vi "Car Wash.vi"() -> ()   [LabVIEW 2025]
uses:
  Controls/Car Wash Indicators.ctl
  Controls/Wash Options.ctl
  Controls/Controls.ctl
panel:
  in  "Start":bool
  out "Elapsed Time":dbl format="%0.2f"
  in  "stop":bool
  out "Wash Entry":bool
  in  "Wash Options":T1
  in  "Car Position Slider":u8(slide) max=3 scale=0.0..4.0
  out "Car Wash Indicators":T2
  # "Entry Console"
  # "Car Wash Display"
  # "Car Position Simulation"
  # "Pre-Soak\nH-P Wash\nL-P Wax\nSpot Free Rinse"
  # "Underbody Wash\nBug Remover"
  # "Tire Shine\nAir Dry"
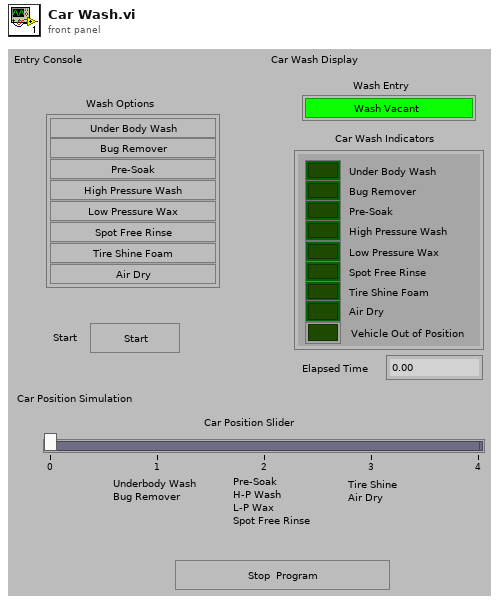
[diagram p1: front panel]
types:
  T1 = typedef "Wash Options.ctl" = cluster{"Underbody Wash":bool, "Bug Remover":bool, "Pre-Soak":bool, "High Pressure Wash":bool, "Low Pressure Wax":bool, "Spot Free Rinse":bool, "Tire Shine Foam":bool, "Air Dry":bool}
  T2 = typedef "Car Wash Indicators.ctl" = cluster{"Under Body Wash":bool, "Bug Remover":bool, "Pre-Soak":bool, "High Pressure Wash":bool, "Low Pressure Wax":bool, "Spot Free Rinse":bool, "Tire Shine Foam":bool, "Air Dry":bool, "Vehicle Out of Position":bool}
  T3 = typedef "Controls.ctl" = enum16{"Initialization", "Wait For Start", "Car Wash Setup", "Under Body Wash", "Bug Remover", "Pre-Soak", "High Pressure Wash", "Low Pressure Wash", "Spot Free Rinse", "Tire Shine Foam", "Air Dry", "Exit"}
  T4 = enum8{"Enabled", "Disabled", "Disabled and Grayed Out"}
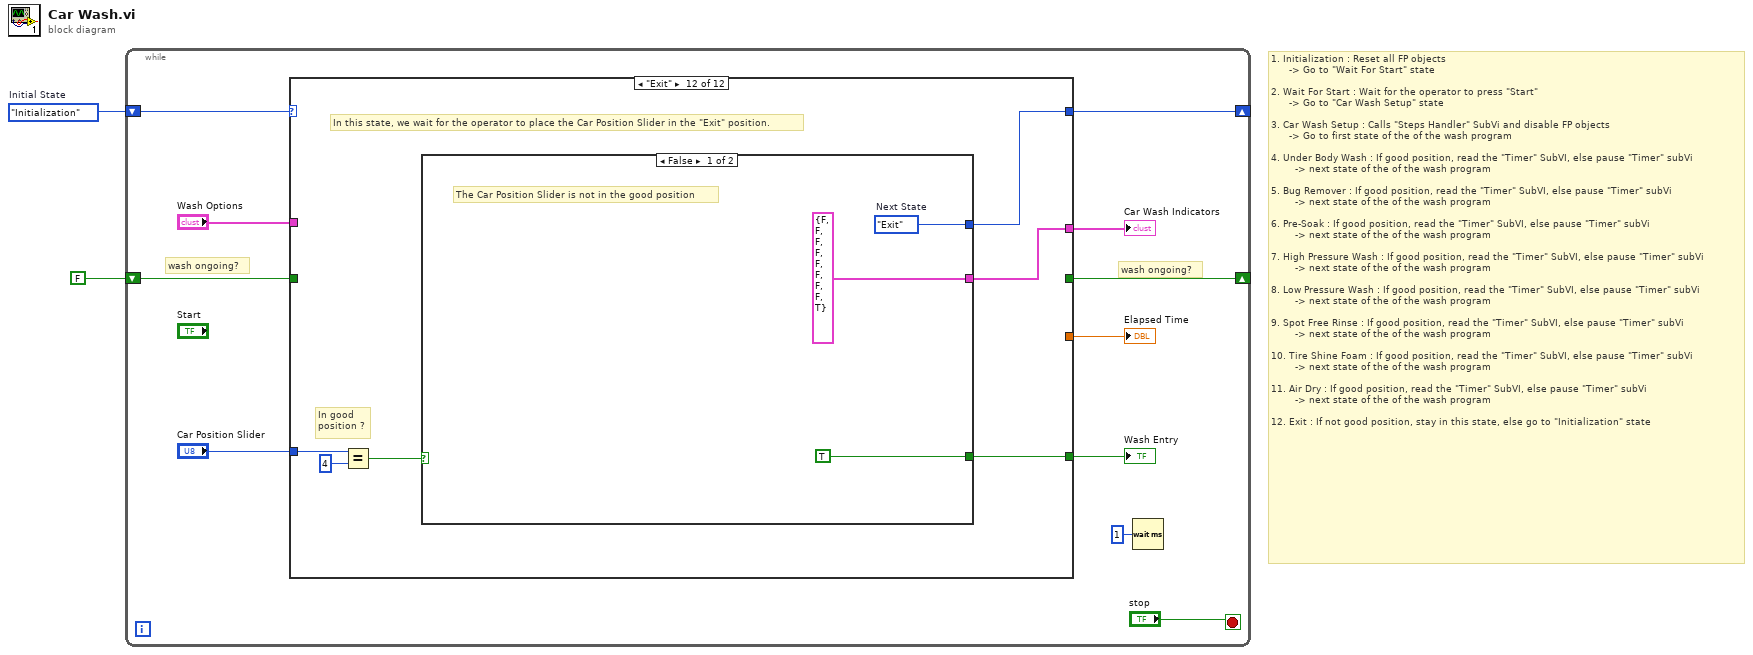
[diagram p0: block diagram]
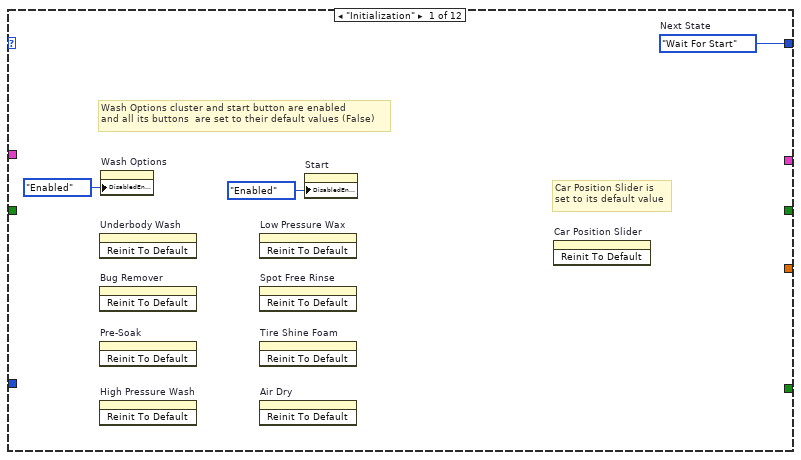
[diagram p2: hidden frame]
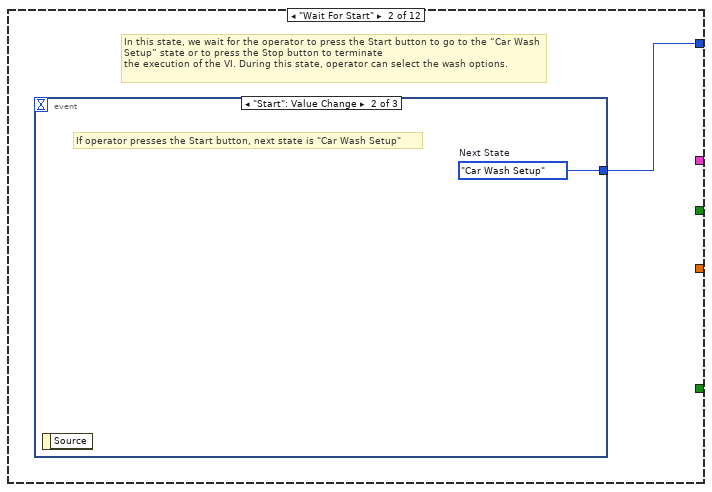
[diagram p3: hidden frame]
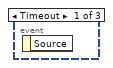
[diagram p4: hidden frame]
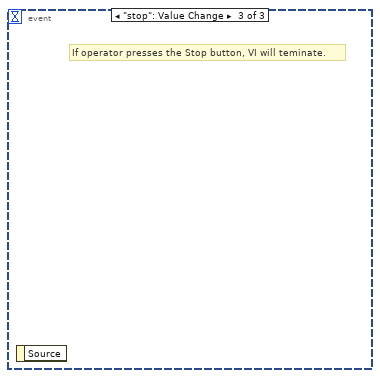
[diagram p5: hidden frame]
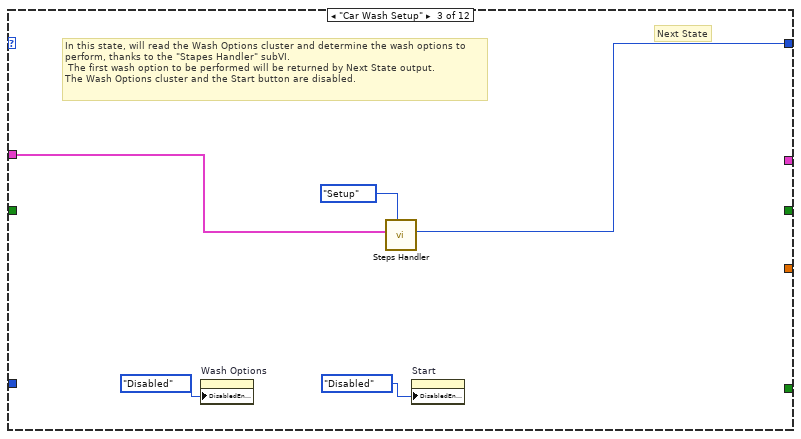
[diagram p6: hidden frame]
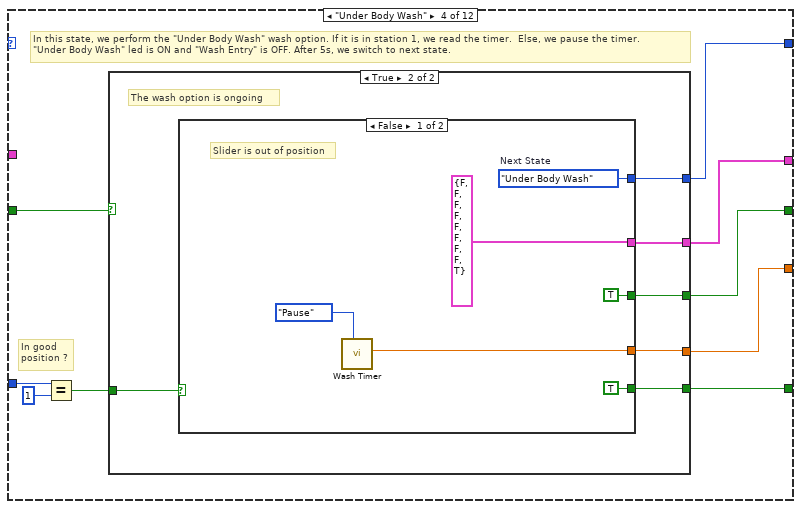
[diagram p7: hidden frame]
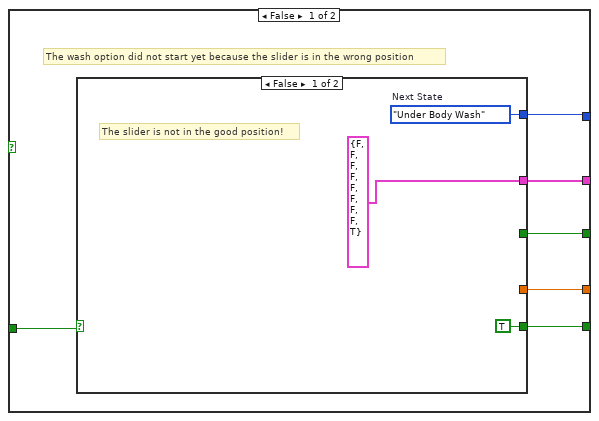
[diagram p8: hidden frame]
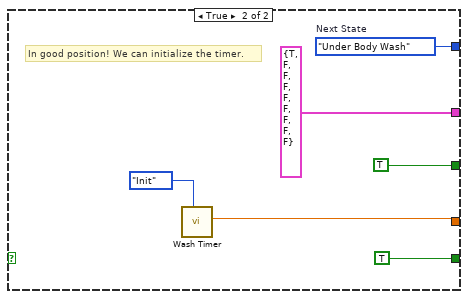
[diagram p9: hidden frame]
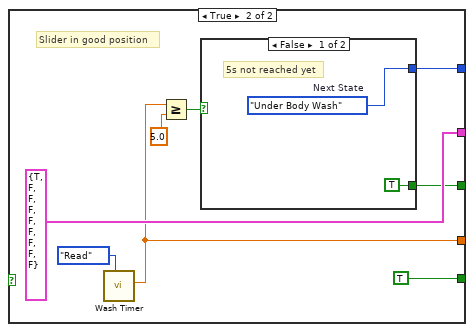
[diagram p10: hidden frame]
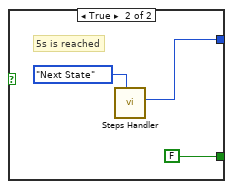
[diagram p11: hidden frame]
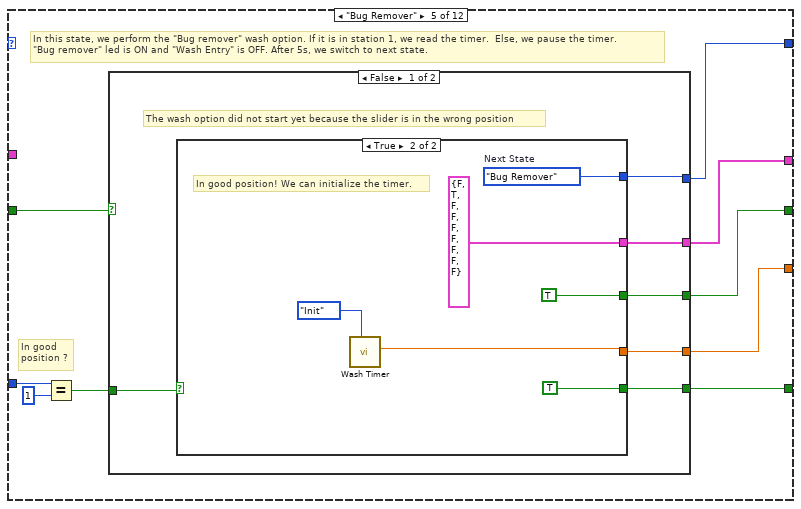
[diagram p12: hidden frame]
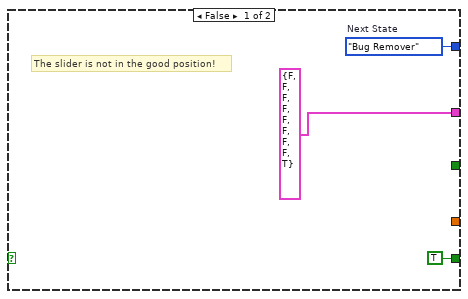
[diagram p13: hidden frame]
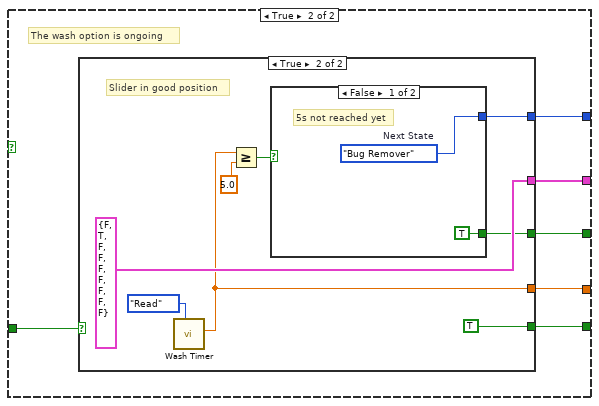
[diagram p14: hidden frame]
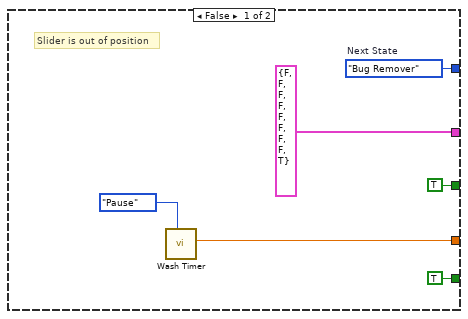
[diagram p15: hidden frame]
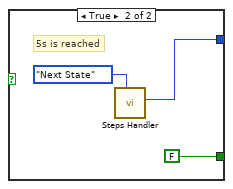
[diagram p16: hidden frame]
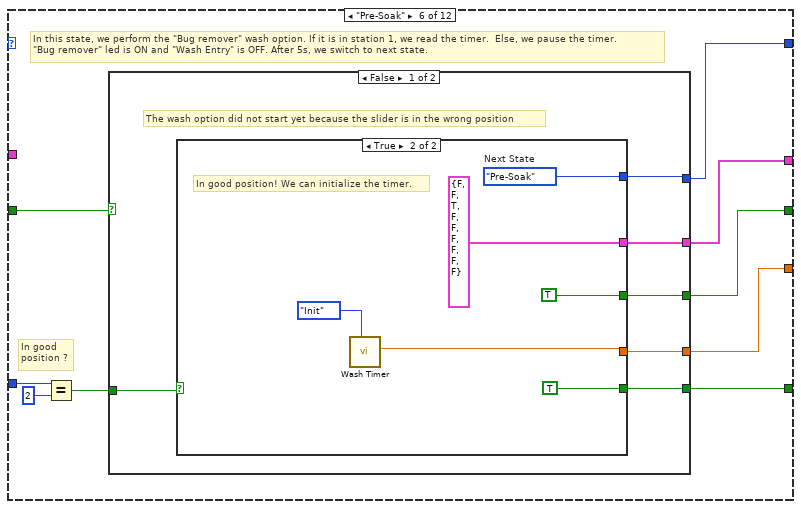
[diagram p17: hidden frame]
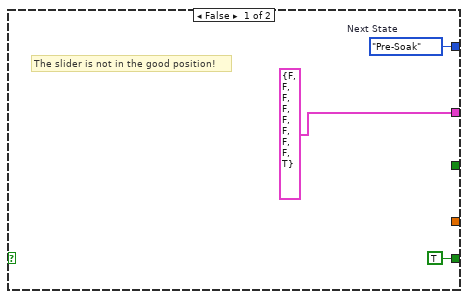
[diagram p18: hidden frame]
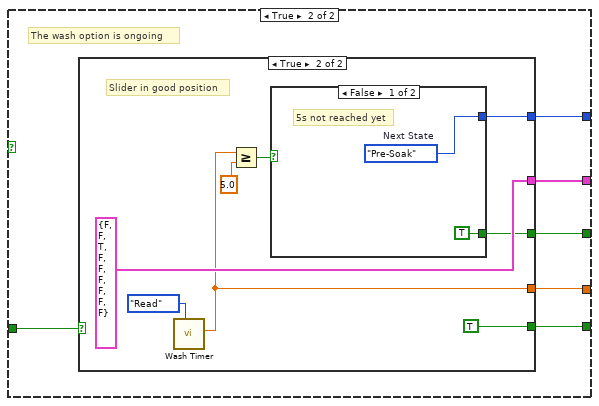
[diagram p19: hidden frame]
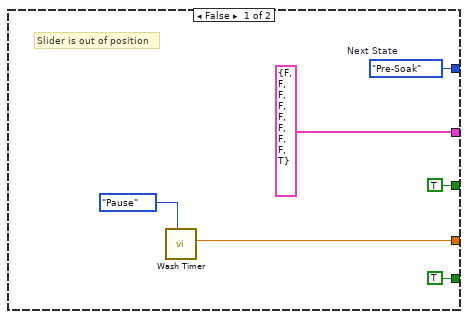
[diagram p20: hidden frame]
diagram:
  w2 = Controls."Initialization"  # Initial State
  # "1. Initialization : Reset all FP objects\n      -> Go to \"Wait For Start\" state\n\n2. Wait For Start : Wait for the operator to press \"Start\"\n      -> Go to \"Car Wash Setup\" state\n\n3. Car Wash Setup : Calls \"Steps Handler\" SubVi and disable FP objects \n      -> Go to first state of the of the wash program \n\n4. Under Body Wash : If good position, read the \"Timer\" SubVI, else pause \"Timer\" subVi\n        -> next state of the of the wash program\n\n5. Bug Remover : If good position, read the \"Timer\" SubVI, else pause \"Timer\" subVi\n        -> next state of the of the wash program\n\n6. Pre-Soak : If good position, read the \"Timer\" SubVI, else pause \"Timer\" subVi\n        -> next state of the of the wash program\n\n7. High Pressure Wash : If good position, read the \"Timer\" SubVI, else pause \"Timer\" subVi\n        -> next state of the of the wash program\n\n8. Low Pressure Wash : If good position, read the \"Timer\" SubVI, else pause \"Timer\" subVi\n        -> next state of the of the wash program\n\n9. Spot Free Rinse : If good position, read the \"Timer\" SubVI, else pause \"Timer\" subVi\n        -> next state of the of the wash program\n\n10. Tire Shine Foam : If good position, read the \"Timer\" SubVI, else pause \"Timer\" subVi\n        -> next state of the of the wash program\n\n11. Air Dry : If good position, read the \"Timer\" SubVI, else pause \"Timer\" subVi\n        -> next state of the of the wash program\n\n12. Exit : If not good position, stay in this state, else go to \"Initialization\" state"
  n1 = while {
    shift-right: [w10] -> _
    shift-left: w2 -> [w13]
    shift-right: [w6] -> _
    shift-left: FALSE -> [w7]
    stop <- "stop" stop-if-true
    # "wash ongoing?"
    # "wash ongoing?"
    n2 = case shown="\"Exit\"" w13 {
      tunnel: [w15 w17 w21 w27 w76 w125 w174 w223 w272 w321 w370 w418] -> w10
      tunnel: "Wash Options" -> [_ _ w22 _ _ _ _ _ _ _ _ _]
      tunnel: "Car Position Slider" -> [_ _ _ w32 w81 w130 w179 w228 w277 w326 w375 w420]
      tunnel: w7 -> [_ _ _ w30 w79 w128 w177 w226 w275 w324 w373 _]
      tunnel: [_ _ _ w28 w77 w126 w175 w224 w273 w322 w371 _] -> w6
      tunnel: [_ _ _ w26 w75 w124 w173 w222 w271 w320 w369 w417] -> w5
      tunnel: [_ _ _ w25 w74 w123 w172 w221 w270 w319 w368 _] -> w4
      tunnel: [_ _ _ w24 w73 w122 w171 w220 w269 w318 w367 w416] -> w3
      frame "Initialization" {
        w15 = Controls."Wait For Start"  # Next State
        # "Car Position Slider is \nset to its default value"
        # "Wash Options cluster and start button are enabled \nand all its buttons  are set to their default values (False)"
        n3 = invoke on="Underbody Wash" class="Bool (strict)" method="Reinit To Default"() -> ()  [unwired: 3 in, 3 out]
        n4 = invoke on="Bug Remover" class="Bool (strict)" method="Reinit To Default"() -> ()  [unwired: 3 in, 3 out]
        n5 = invoke on="Pre-Soak" class="Bool (strict)" method="Reinit To Default"() -> ()  [unwired: 3 in, 3 out]
        n6 = invoke on="High Pressure Wash" class="Bool (strict)" method="Reinit To Default"() -> ()  [unwired: 3 in, 3 out]
        n7 = property on="Wash Options" class="Clust (strict)"("DisabledEnum"=T4."Enabled" ("Disabled")) -> ()  [unwired: 2 in, 2 out]
        n8 = invoke on="Low Pressure Wax" class="Bool (strict)" method="Reinit To Default"() -> ()  [unwired: 3 in, 3 out]
        n9 = invoke on="Spot Free Rinse" class="Bool (strict)" method="Reinit To Default"() -> ()  [unwired: 3 in, 3 out]
        n10 = invoke on="Tire Shine Foam" class="Bool (strict)" method="Reinit To Default"() -> ()  [unwired: 3 in, 3 out]
        n11 = invoke on="Air Dry" class="Bool (strict)" method="Reinit To Default"() -> ()  [unwired: 3 in, 3 out]
        n12 = property on="Start" class="Bool"("DisabledEnum"=T4."Enabled" ("Disabled")) -> ()  [unwired: 2 in, 2 out]
        n13 = invoke on="Car Position Slider" class="Slide (strict)" method="Reinit To Default"() -> ()  [unwired: 3 in, 3 out]
      }
      frame "Wait For Start" {
        # "In this state, we wait for the operator to press the Start button to go to the “Car Wash Setup” state or to press the Stop button to terminate \nthe execution of the VI. During this state, operator can select the wash options."
        n14 = event shown="[1] \"Start\": Value Change" {
          selector: _ -> [_ _ _]
          dyn-events: _ -> [_ _ _]
          timeout: _ -> [_ _ _]
          tunnel: [_ w18 _] -> w17
          event Timeout {
            n15 = event-data() -> ()  [unwired: 1 in, 1 out]
          }
          event "Start": Value Change {
            w18 = Controls."Car Wash Setup"  # Next State
            # "If operator presses the Start button, next state is \"Car Wash Setup\""
            n16 = event-data() -> ()  [unwired: 1 in, 1 out]
          }
          event "stop": Value Change {
            # "If operator presses the Stop button, VI will teminate."
            n17 = event-data() -> ()  [unwired: 1 in, 1 out]
          }
        }
      }
      frame "Car Wash Setup" {
        # "In this state, will read the Wash Options cluster and determine the wash options to perform, thanks to the \"Stapes Handler\" subVI.\n The first wash option to be performed will be returned by Next State output.\nThe Wash Options cluster and the Start button are disabled."
        # "Next State"
        n18 = property on="Wash Options" class="Clust (strict)"("DisabledEnum"=T4."Disabled" ("Disabled")) -> ()  [unwired: 2 in, 2 out]
        n19 = call "Steps Handler.vi"("Operation"=enum16{"Setup", "Next State"}."Setup", "Wash Options"=w22) -> ("Next State"=w21:T3)  [unwired: 9 in]
        n20 = property on="Start" class="Bool"("DisabledEnum"=T4."Disabled" ("Disabled")) -> ()  [unwired: 2 in, 2 out]
      }
      frame "Under Body Wash" {
        # "In good \nposition ?"
        # "In this state, we perform the \"Under Body Wash\" wash option. If it is in station 1, we read the timer.  Else, we pause the timer. \n\"Under Body Wash\" led is ON and \"Wash Entry\" is OFF. After 5s, we switch to next state."
        n21 = Equal?(x=w32, y=u8 1) -> (x = y?=w29:bool)
        n22 = case shown="True" w30 {
          tunnel: w29 -> [w38 w53]
          tunnel: [w37 w48] -> w28
          tunnel: [w36 w49] -> w27
          tunnel: [w35 w50] -> w26
          tunnel: [w34 w52] -> w25
          tunnel: [w33 w51] -> w24
          frame False {
            # "The wash option did not start yet because the slider is in the wrong position"
            n23 = case shown="False" w38 {
              tunnel: [_ TRUE] -> w37
              tunnel: [w41 w46] -> w36
              tunnel: [T2 {"Under Body Wash"=FALSE, "Bug Remover"=FALSE, "Pre-Soak"=FALSE, "High Pressure Wash"=FALSE, "Low Pressure Wax"=FALSE, "Spot Free Rinse"=FALSE, "Tire Shine Foam"=FALSE, "Air Dry"=FALSE, "Vehicle Out of Position"=TRUE} ("Car Wash Indicators") T2 {"Under Body Wash"=TRUE, "Bug Remover"=FALSE, "Pre-Soak"=FALSE, "High Pressure Wash"=FALSE, "Low Pressure Wax"=FALSE, "Spot Free Rinse"=FALSE, "Tire Shine Foam"=FALSE, "Air Dry"=FALSE, "Vehicle Out of Position"=FALSE} ("Car Wash Indicators")] -> w35
              tunnel: [_ w43] -> w34
              tunnel: [TRUE TRUE] -> w33
              frame False {
                w41 = Controls."Under Body Wash"  # Next State
                # "The slider is not in the good position!"
              }
              frame True {
                w46 = Controls."Under Body Wash"  # Next State
                # "In good position! We can initialize the timer."
                n24 = call "Wash Timer.vi"("Operation"=enum16{"Init", "Read", "Pause"}."Init") -> ("count"=w43:dbl)  [unwired: 10 in]
              }
            }
          }
          frame True {
            # "The wash option is ongoing"
            n25 = case shown="False" w53 {
              tunnel: [w58 w64] -> w52
              tunnel: [TRUE TRUE] -> w51
              tunnel: [T2 {"Under Body Wash"=FALSE, "Bug Remover"=FALSE, "Pre-Soak"=FALSE, "High Pressure Wash"=FALSE, "Low Pressure Wax"=FALSE, "Spot Free Rinse"=FALSE, "Tire Shine Foam"=FALSE, "Air Dry"=FALSE, "Vehicle Out of Position"=TRUE} ("Car Wash Indicators") T2 {"Under Body Wash"=TRUE, "Bug Remover"=FALSE, "Pre-Soak"=FALSE, "High Pressure Wash"=FALSE, "Low Pressure Wax"=FALSE, "Spot Free Rinse"=FALSE, "Tire Shine Foam"=FALSE, "Air Dry"=FALSE, "Vehicle Out of Position"=FALSE} ("Car Wash Indicators")] -> w50
              tunnel: [w57 w61] -> w49
              tunnel: [TRUE w60] -> w48
              frame False {
                w57 = Controls."Under Body Wash"  # Next State
                # "Slider is out of position"
                n26 = call "Wash Timer.vi"("Operation"=enum16{"Init", "Read", "Pause"}."Pause") -> ("count"=w58:dbl)  [unwired: 10 in]
              }
              frame True {
                # "Slider in good position"
                n27 = call "Wash Timer.vi"("Operation"=enum16{"Init", "Read", "Pause"}."Read") -> ("count"=w64:dbl)  [unwired: 10 in]
                n28 = Greater Or Equal?(x=w64, y=5.0) -> (x >= y?=w62:bool)
                n29 = case shown="False" w62 {
                  tunnel: [w69 w71] -> w61
                  tunnel: [TRUE FALSE] -> w60
                  frame False {
                    w69 = Controls."Under Body Wash"  # Next State
                    # "5s not reached yet"
                  }
                  frame True {
                    # "5s is reached"
                    n30 = call "Steps Handler.vi"("Operation"=enum16{"Setup", "Next State"}."Next State") -> ("Next State"=w71:T3)  [unwired: 10 in]
                  }
                }
              }
            }
          }
        }
      }
      frame "Bug Remover" {
        # "In good \nposition ?"
        # "In this state, we perform the \"Bug remover\" wash option. If it is in station 1, we read the timer.  Else, we pause the timer. \n\"Bug remover\" led is ON and \"Wash Entry\" is OFF. After 5s, we switch to next state."
        n31 = Equal?(x=w81, y=u8 1) -> (x = y?=w78:bool)
        n32 = case shown="False" w79 {
          tunnel: w78 -> [w87 w102]
          tunnel: [w86 w97] -> w77
          tunnel: [w85 w98] -> w76
          tunnel: [w84 w99] -> w75
          tunnel: [w83 w101] -> w74
          tunnel: [w82 w100] -> w73
          frame False {
            # "The wash option did not start yet because the slider is in the wrong position"
            n33 = case shown="True" w87 {
              tunnel: [_ TRUE] -> w86
              tunnel: [w90 w95] -> w85
              tunnel: [T2 {"Under Body Wash"=FALSE, "Bug Remover"=FALSE, "Pre-Soak"=FALSE, "High Pressure Wash"=FALSE, "Low Pressure Wax"=FALSE, "Spot Free Rinse"=FALSE, "Tire Shine Foam"=FALSE, "Air Dry"=FALSE, "Vehicle Out of Position"=TRUE} ("Car Wash Indicators") T2 {"Under Body Wash"=FALSE, "Bug Remover"=TRUE, "Pre-Soak"=FALSE, "High Pressure Wash"=FALSE, "Low Pressure Wax"=FALSE, "Spot Free Rinse"=FALSE, "Tire Shine Foam"=FALSE, "Air Dry"=FALSE, "Vehicle Out of Position"=FALSE} ("Car Wash Indicators")] -> w84
              tunnel: [_ w92] -> w83
              tunnel: [TRUE TRUE] -> w82
              frame False {
                w90 = Controls."Bug Remover"  # Next State
                # "The slider is not in the good position!"
              }
              frame True {
                w95 = Controls."Bug Remover"  # Next State
                # "In good position! We can initialize the timer."
                n34 = call "Wash Timer.vi"("Operation"=enum16{"Init", "Read", "Pause"}."Init") -> ("count"=w92:dbl)  [unwired: 10 in]
              }
            }
          }
          frame True {
            # "The wash option is ongoing"
            n35 = case shown="True" w102 {
              tunnel: [w107 w113] -> w101
              tunnel: [TRUE TRUE] -> w100
              tunnel: [T2 {"Under Body Wash"=FALSE, "Bug Remover"=FALSE, "Pre-Soak"=FALSE, "High Pressure Wash"=FALSE, "Low Pressure Wax"=FALSE, "Spot Free Rinse"=FALSE, "Tire Shine Foam"=FALSE, "Air Dry"=FALSE, "Vehicle Out of Position"=TRUE} ("Car Wash Indicators") T2 {"Under Body Wash"=FALSE, "Bug Remover"=TRUE, "Pre-Soak"=FALSE, "High Pressure Wash"=FALSE, "Low Pressure Wax"=FALSE, "Spot Free Rinse"=FALSE, "Tire Shine Foam"=FALSE, "Air Dry"=FALSE, "Vehicle Out of Position"=FALSE} ("Car Wash Indicators")] -> w99
              tunnel: [w106 w110] -> w98
              tunnel: [TRUE w109] -> w97
              frame False {
                w106 = Controls."Bug Remover"  # Next State
                # "Slider is out of position"
                n36 = call "Wash Timer.vi"("Operation"=enum16{"Init", "Read", "Pause"}."Pause") -> ("count"=w107:dbl)  [unwired: 10 in]
              }
              frame True {
                # "Slider in good position"
                n37 = call "Wash Timer.vi"("Operation"=enum16{"Init", "Read", "Pause"}."Read") -> ("count"=w113:dbl)  [unwired: 10 in]
                n38 = Greater Or Equal?(x=w113, y=5.0) -> (x >= y?=w111:bool)
                n39 = case shown="False" w111 {
                  tunnel: [w118 w120] -> w110
                  tunnel: [TRUE FALSE] -> w109
                  frame False {
                    w118 = Controls."Bug Remover"  # Next State
                    # "5s not reached yet"
                  }
                  frame True {
                    # "5s is reached"
                    n40 = call "Steps Handler.vi"("Operation"=enum16{"Setup", "Next State"}."Next State") -> ("Next State"=w120:T3)  [unwired: 10 in]
                  }
                }
              }
            }
          }
        }
      }
      frame "Pre-Soak" {
        # "In good \nposition ?"
        # "In this state, we perform the \"Bug remover\" wash option. If it is in station 1, we read the timer.  Else, we pause the timer. \n\"Bug remover\" led is ON and \"Wash Entry\" is OFF. After 5s, we switch to next state."
        n41 = Equal?(x=w130, y=u8 2) -> (x = y?=w127:bool)
        n42 = case shown="False" w128 {
          tunnel: w127 -> [w136 w151]
          tunnel: [w135 w146] -> w126
          tunnel: [w134 w147] -> w125
          tunnel: [w133 w148] -> w124
          tunnel: [w132 w150] -> w123
          tunnel: [w131 w149] -> w122
          frame False {
            # "The wash option did not start yet because the slider is in the wrong position"
            n43 = case shown="True" w136 {
              tunnel: [_ TRUE] -> w135
              tunnel: [w139 w144] -> w134
              tunnel: [T2 {"Under Body Wash"=FALSE, "Bug Remover"=FALSE, "Pre-Soak"=FALSE, "High Pressure Wash"=FALSE, "Low Pressure Wax"=FALSE, "Spot Free Rinse"=FALSE, "Tire Shine Foam"=FALSE, "Air Dry"=FALSE, "Vehicle Out of Position"=TRUE} ("Car Wash Indicators") T2 {"Under Body Wash"=FALSE, "Bug Remover"=FALSE, "Pre-Soak"=TRUE, "High Pressure Wash"=FALSE, "Low Pressure Wax"=FALSE, "Spot Free Rinse"=FALSE, "Tire Shine Foam"=FALSE, "Air Dry"=FALSE, "Vehicle Out of Position"=FALSE} ("Car Wash Indicators")] -> w133
              tunnel: [_ w141] -> w132
              tunnel: [TRUE TRUE] -> w131
              frame False {
                w139 = Controls."Pre-Soak"  # Next State
                # "The slider is not in the good position!"
              }
              frame True {
                w144 = Controls."Pre-Soak"  # Next State
                # "In good position! We can initialize the timer."
                n44 = call "Wash Timer.vi"("Operation"=enum16{"Init", "Read", "Pause"}."Init") -> ("count"=w141:dbl)  [unwired: 10 in]
              }
            }
          }
          frame True {
            # "The wash option is ongoing"
            n45 = case shown="True" w151 {
              tunnel: [w156 w162] -> w150
              tunnel: [TRUE TRUE] -> w149
              tunnel: [T2 {"Under Body Wash"=FALSE, "Bug Remover"=FALSE, "Pre-Soak"=FALSE, "High Pressure Wash"=FALSE, "Low Pressure Wax"=FALSE, "Spot Free Rinse"=FALSE, "Tire Shine Foam"=FALSE, "Air Dry"=FALSE, "Vehicle Out of Position"=TRUE} ("Car Wash Indicators") T2 {"Under Body Wash"=FALSE, "Bug Remover"=FALSE, "Pre-Soak"=TRUE, "High Pressure Wash"=FALSE, "Low Pressure Wax"=FALSE, "Spot Free Rinse"=FALSE, "Tire Shine Foam"=FALSE, "Air Dry"=FALSE, "Vehicle Out of Position"=FALSE} ("Car Wash Indicators")] -> w148
              tunnel: [w155 w159] -> w147
              tunnel: [TRUE w158] -> w146
              frame False {
                w155 = Controls."Pre-Soak"  # Next State
                # "Slider is out of position"
                n46 = call "Wash Timer.vi"("Operation"=enum16{"Init", "Read", "Pause"}."Pause") -> ("count"=w156:dbl)  [unwired: 10 in]
              }
              frame True {
                # "Slider in good position"
                n47 = call "Wash Timer.vi"("Operation"=enum16{"Init", "Read", "Pause"}."Read") -> ("count"=w162:dbl)  [unwired: 10 in]
                n48 = Greater Or Equal?(x=w162, y=5.0) -> (x >= y?=w160:bool)
                n49 = case shown="False" w160 {
                  tunnel: [w167 w169] -> w159
                  tunnel: [TRUE FALSE] -> w158
                  frame False {
                    w167 = Controls."Pre-Soak"  # Next State
                    # "5s not reached yet"
                  }
                  frame True {
                    # "5s is reached"
                    n50 = call "Steps Handler.vi"("Operation"=enum16{"Setup", "Next State"}."Next State") -> ("Next State"=w169:T3)  [unwired: 10 in]
                  }
                }
              }
            }
          }
        }
      }
      frame "High Pressure Wash" {
        # "In good \nposition ?"
        # "In this state, we perform the \"Bug remover\" wash option. If it is in station 1, we read the timer.  Else, we pause the timer. \n\"Bug remover\" led is ON and \"Wash Entry\" is OFF. After 5s, we switch to next state."
        n51 = Equal?(x=w179, y=u8 2) -> (x = y?=w176:bool)
        n52 = case shown="False" w177 {
          tunnel: w176 -> [w185 w200]
          tunnel: [w184 w195] -> w175
          tunnel: [w183 w196] -> w174
          tunnel: [w182 w197] -> w173
          tunnel: [w181 w199] -> w172
          tunnel: [w180 w198] -> w171
          frame False {
            # "The wash option did not start yet because the slider is in the wrong position"
            n53 = case shown="False" w185 {
              tunnel: [_ TRUE] -> w184
              tunnel: [w188 w193] -> w183
              tunnel: [T2 {"Under Body Wash"=FALSE, "Bug Remover"=FALSE, "Pre-Soak"=FALSE, "High Pressure Wash"=FALSE, "Low Pressure Wax"=FALSE, "Spot Free Rinse"=FALSE, "Tire Shine Foam"=FALSE, "Air Dry"=FALSE, "Vehicle Out of Position"=TRUE} ("Car Wash Indicators") T2 {"Under Body Wash"=FALSE, "Bug Remover"=FALSE, "Pre-Soak"=FALSE, "High Pressure Wash"=TRUE, "Low Pressure Wax"=FALSE, "Spot Free Rinse"=FALSE, "Tire Shine Foam"=FALSE, "Air Dry"=FALSE, "Vehicle Out of Position"=FALSE} ("Car Wash Indicators")] -> w182
              tunnel: [_ w190] -> w181
              tunnel: [TRUE TRUE] -> w180
              frame False {
                w188 = Controls."High Pressure Wash"  # Next State
                # "The slider is not in the good position!"
              }
              frame True {
                w193 = Controls."High Pressure Wash"  # Next State
                # "In good position! We can initialize the timer."
                n54 = call "Wash Timer.vi"("Operation"=enum16{"Init", "Read", "Pause"}."Init") -> ("count"=w190:dbl)  [unwired: 10 in]
              }
            }
          }
          frame True {
            # "The wash option is ongoing"
            n55 = case shown="False" w200 {
              tunnel: [w205 w211] -> w199
              tunnel: [TRUE TRUE] -> w198
              tunnel: [T2 {"Under Body Wash"=FALSE, "Bug Remover"=FALSE, "Pre-Soak"=FALSE, "High Pressure Wash"=FALSE, "Low Pressure Wax"=FALSE, "Spot Free Rinse"=FALSE, "Tire Shine Foam"=FALSE, "Air Dry"=FALSE, "Vehicle Out of Position"=TRUE} ("Car Wash Indicators") T2 {"Under Body Wash"=FALSE, "Bug Remover"=FALSE, "Pre-Soak"=FALSE, "High Pressure Wash"=TRUE, "Low Pressure Wax"=FALSE, "Spot Free Rinse"=FALSE, "Tire Shine Foam"=FALSE, "Air Dry"=FALSE, "Vehicle Out of Position"=FALSE} ("Car Wash Indicators")] -> w197
              tunnel: [w204 w208] -> w196
              tunnel: [TRUE w207] -> w195
              frame False {
                w204 = Controls."High Pressure Wash"  # Next State
                # "Slider is out of position"
                n56 = call "Wash Timer.vi"("Operation"=enum16{"Init", "Read", "Pause"}."Pause") -> ("count"=w205:dbl)  [unwired: 10 in]
              }
              frame True {
                # "Slider in good position"
                n57 = call "Wash Timer.vi"("Operation"=enum16{"Init", "Read", "Pause"}."Read") -> ("count"=w211:dbl)  [unwired: 10 in]
                n58 = Greater Or Equal?(x=w211, y=5.0) -> (x >= y?=w209:bool)
                n59 = case shown="False" w209 {
                  tunnel: [w216 w218] -> w208
                  tunnel: [TRUE FALSE] -> w207
                  frame False {
                    w216 = Controls."High Pressure Wash"  # Next State
                    # "5s not reached yet"
                  }
                  frame True {
                    # "5s is reached"
                    n60 = call "Steps Handler.vi"("Operation"=enum16{"Setup", "Next State"}."Next State") -> ("Next State"=w218:T3)  [unwired: 10 in]
                  }
                }
              }
            }
          }
        }
      }
      frame "Low Pressure Wash" {
        # "In good \nposition ?"
        # "In this state, we perform the \"Bug remover\" wash option. If it is in station 1, we read the timer.  Else, we pause the timer. \n\"Bug remover\" led is ON and \"Wash Entry\" is OFF. After 5s, we switch to next state."
        n61 = Equal?(x=w228, y=u8 2) -> (x = y?=w225:bool)
        n62 = case shown="True" w226 {
          tunnel: w225 -> [w234 w249]
          tunnel: [w233 w244] -> w224
          tunnel: [w232 w245] -> w223
          tunnel: [w231 w246] -> w222
          tunnel: [w230 w248] -> w221
          tunnel: [w229 w247] -> w220
          frame False {
            # "The wash option did not start yet because the slider is in the wrong position"
            n63 = case shown="True" w234 {
              tunnel: [_ TRUE] -> w233
              tunnel: [w237 w242] -> w232
              tunnel: [T2 {"Under Body Wash"=FALSE, "Bug Remover"=FALSE, "Pre-Soak"=FALSE, "High Pressure Wash"=FALSE, "Low Pressure Wax"=FALSE, "Spot Free Rinse"=FALSE, "Tire Shine Foam"=FALSE, "Air Dry"=FALSE, "Vehicle Out of Position"=TRUE} ("Car Wash Indicators") T2 {"Under Body Wash"=FALSE, "Bug Remover"=FALSE, "Pre-Soak"=FALSE, "High Pressure Wash"=FALSE, "Low Pressure Wax"=TRUE, "Spot Free Rinse"=FALSE, "Tire Shine Foam"=FALSE, "Air Dry"=FALSE, "Vehicle Out of Position"=FALSE} ("Car Wash Indicators")] -> w231
              tunnel: [_ w239] -> w230
              tunnel: [TRUE TRUE] -> w229
              frame False {
                w237 = Controls."Low Pressure Wash"  # Next State
                # "The slider is not in the good position!"
              }
              frame True {
                w242 = Controls."Low Pressure Wash"  # Next State
                # "In good position! We can initialize the timer."
                n64 = call "Wash Timer.vi"("Operation"=enum16{"Init", "Read", "Pause"}."Init") -> ("count"=w239:dbl)  [unwired: 10 in]
              }
            }
          }
          frame True {
            # "The wash option is ongoing"
            n65 = case shown="True" w249 {
              tunnel: [w254 w260] -> w248
              tunnel: [TRUE TRUE] -> w247
              tunnel: [T2 {"Under Body Wash"=FALSE, "Bug Remover"=FALSE, "Pre-Soak"=FALSE, "High Pressure Wash"=FALSE, "Low Pressure Wax"=FALSE, "Spot Free Rinse"=FALSE, "Tire Shine Foam"=FALSE, "Air Dry"=FALSE, "Vehicle Out of Position"=TRUE} ("Car Wash Indicators") T2 {"Under Body Wash"=FALSE, "Bug Remover"=FALSE, "Pre-Soak"=FALSE, "High Pressure Wash"=FALSE, "Low Pressure Wax"=TRUE, "Spot Free Rinse"=FALSE, "Tire Shine Foam"=FALSE, "Air Dry"=FALSE, "Vehicle Out of Position"=FALSE} ("Car Wash Indicators")] -> w246
              tunnel: [w253 w257] -> w245
              tunnel: [TRUE w256] -> w244
              frame False {
                w253 = Controls."Low Pressure Wash"  # Next State
                # "Slider is out of position"
                n66 = call "Wash Timer.vi"("Operation"=enum16{"Init", "Read", "Pause"}."Pause") -> ("count"=w254:dbl)  [unwired: 10 in]
              }
              frame True {
                # "Slider in good position"
                n67 = call "Wash Timer.vi"("Operation"=enum16{"Init", "Read", "Pause"}."Read") -> ("count"=w260:dbl)  [unwired: 10 in]
                n68 = Greater Or Equal?(x=w260, y=5.0) -> (x >= y?=w258:bool)
                n69 = case shown="False" w258 {
                  tunnel: [w265 w267] -> w257
                  tunnel: [TRUE FALSE] -> w256
                  frame False {
                    w265 = Controls."Low Pressure Wash"  # Next State
                    # "5s not reached yet"
                  }
                  frame True {
                    # "5s is reached"
                    n70 = call "Steps Handler.vi"("Operation"=enum16{"Setup", "Next State"}."Next State") -> ("Next State"=w267:T3)  [unwired: 10 in]
                  }
                }
              }
            }
          }
        }
      }
      frame "Spot Free Rinse" {
        # "In good \nposition ?"
        # "In this state, we perform the \"Bug remover\" wash option. If it is in station 1, we read the timer.  Else, we pause the timer. \n\"Bug remover\" led is ON and \"Wash Entry\" is OFF. After 5s, we switch to next state."
        n71 = Equal?(x=w277, y=u8 2) -> (x = y?=w274:bool)
        n72 = case shown="True" w275 {
          tunnel: w274 -> [w283 w298]
          tunnel: [w282 w293] -> w273
          tunnel: [w281 w294] -> w272
          tunnel: [w280 w295] -> w271
          tunnel: [w279 w297] -> w270
          tunnel: [w278 w296] -> w269
          frame False {
            # "The wash option did not start yet because the slider is in the wrong position"
            n73 = case shown="True" w283 {
              tunnel: [_ TRUE] -> w282
              tunnel: [w286 w291] -> w281
              tunnel: [T2 {"Under Body Wash"=FALSE, "Bug Remover"=FALSE, "Pre-Soak"=FALSE, "High Pressure Wash"=FALSE, "Low Pressure Wax"=FALSE, "Spot Free Rinse"=FALSE, "Tire Shine Foam"=FALSE, "Air Dry"=FALSE, "Vehicle Out of Position"=TRUE} ("Car Wash Indicators") T2 {"Under Body Wash"=FALSE, "Bug Remover"=FALSE, "Pre-Soak"=FALSE, "High Pressure Wash"=FALSE, "Low Pressure Wax"=FALSE, "Spot Free Rinse"=TRUE, "Tire Shine Foam"=FALSE, "Air Dry"=FALSE, "Vehicle Out of Position"=FALSE} ("Car Wash Indicators")] -> w280
              tunnel: [_ w288] -> w279
              tunnel: [TRUE TRUE] -> w278
              frame False {
                w286 = Controls."Spot Free Rinse"  # Next State
                # "The slider is not in the good position!"
              }
              frame True {
                w291 = Controls."Spot Free Rinse"  # Next State
                # "In good position! We can initialize the timer."
                n74 = call "Wash Timer.vi"("Operation"=enum16{"Init", "Read", "Pause"}."Init") -> ("count"=w288:dbl)  [unwired: 10 in]
              }
            }
          }
          frame True {
            # "The wash option is ongoing"
            n75 = case shown="True" w298 {
              tunnel: [w303 w309] -> w297
              tunnel: [TRUE TRUE] -> w296
              tunnel: [T2 {"Under Body Wash"=FALSE, "Bug Remover"=FALSE, "Pre-Soak"=FALSE, "High Pressure Wash"=FALSE, "Low Pressure Wax"=FALSE, "Spot Free Rinse"=FALSE, "Tire Shine Foam"=FALSE, "Air Dry"=FALSE, "Vehicle Out of Position"=TRUE} ("Car Wash Indicators") T2 {"Under Body Wash"=FALSE, "Bug Remover"=FALSE, "Pre-Soak"=FALSE, "High Pressure Wash"=FALSE, "Low Pressure Wax"=FALSE, "Spot Free Rinse"=TRUE, "Tire Shine Foam"=FALSE, "Air Dry"=FALSE, "Vehicle Out of Position"=FALSE} ("Car Wash Indicators")] -> w295
              tunnel: [w302 w306] -> w294
              tunnel: [TRUE w305] -> w293
              frame False {
                w302 = Controls."Spot Free Rinse"  # Next State
                # "Slider is out of position"
                n76 = call "Wash Timer.vi"("Operation"=enum16{"Init", "Read", "Pause"}."Pause") -> ("count"=w303:dbl)  [unwired: 10 in]
              }
              frame True {
                # "Slider in good position"
                n77 = call "Wash Timer.vi"("Operation"=enum16{"Init", "Read", "Pause"}."Read") -> ("count"=w309:dbl)  [unwired: 10 in]
                n78 = Greater Or Equal?(x=w309, y=5.0) -> (x >= y?=w307:bool)
                n79 = case shown="True" w307 {
                  tunnel: [w314 w316] -> w306
                  tunnel: [TRUE FALSE] -> w305
                  frame False {
                    w314 = Controls."Spot Free Rinse"  # Next State
                    # "5s not reached yet"
                  }
                  frame True {
                    # "5s is reached"
                    n80 = call "Steps Handler.vi"("Operation"=enum16{"Setup", "Next State"}."Next State") -> ("Next State"=w316:T3)  [unwired: 10 in]
                  }
                }
              }
            }
          }
        }
      }
      frame "Tire Shine Foam" {
        # "In good \nposition ?"
        # "In this state, we perform the \"Bug remover\" wash option. If it is in station 1, we read the timer.  Else, we pause the timer. \n\"Bug remover\" led is ON and \"Wash Entry\" is OFF. After 5s, we switch to next state."
        n81 = Equal?(x=w326, y=u8 3) -> (x = y?=w323:bool)
        n82 = case shown="False" w324 {
          tunnel: w323 -> [w332 w347]
          tunnel: [w331 w342] -> w322
          tunnel: [w330 w343] -> w321
          tunnel: [w329 w344] -> w320
          tunnel: [w328 w346] -> w319
          tunnel: [w327 w345] -> w318
          frame False {
            # "The wash option did not start yet because the slider is in the wrong position"
            n83 = case shown="False" w332 {
              tunnel: [_ TRUE] -> w331
              tunnel: [w335 w340] -> w330
              tunnel: [T2 {"Under Body Wash"=FALSE, "Bug Remover"=FALSE, "Pre-Soak"=FALSE, "High Pressure Wash"=FALSE, "Low Pressure Wax"=FALSE, "Spot Free Rinse"=FALSE, "Tire Shine Foam"=FALSE, "Air Dry"=FALSE, "Vehicle Out of Position"=TRUE} ("Car Wash Indicators") T2 {"Under Body Wash"=FALSE, "Bug Remover"=FALSE, "Pre-Soak"=FALSE, "High Pressure Wash"=FALSE, "Low Pressure Wax"=FALSE, "Spot Free Rinse"=FALSE, "Tire Shine Foam"=TRUE, "Air Dry"=FALSE, "Vehicle Out of Position"=FALSE} ("Car Wash Indicators")] -> w329
              tunnel: [_ w337] -> w328
              tunnel: [TRUE TRUE] -> w327
              frame False {
                w335 = Controls."Tire Shine Foam"  # Next State
                # "The slider is not in the good position!"
              }
              frame True {
                w340 = Controls."Tire Shine Foam"  # Next State
                # "In good position! We can initialize the timer."
                n84 = call "Wash Timer.vi"("Operation"=enum16{"Init", "Read", "Pause"}."Init") -> ("count"=w337:dbl)  [unwired: 10 in]
              }
            }
          }
          frame True {
            # "The wash option is ongoing"
            n85 = case shown="False" w347 {
              tunnel: [w352 w358] -> w346
              tunnel: [TRUE TRUE] -> w345
              tunnel: [T2 {"Under Body Wash"=FALSE, "Bug Remover"=FALSE, "Pre-Soak"=FALSE, "High Pressure Wash"=FALSE, "Low Pressure Wax"=FALSE, "Spot Free Rinse"=FALSE, "Tire Shine Foam"=FALSE, "Air Dry"=FALSE, "Vehicle Out of Position"=TRUE} ("Car Wash Indicators") T2 {"Under Body Wash"=FALSE, "Bug Remover"=FALSE, "Pre-Soak"=FALSE, "High Pressure Wash"=FALSE, "Low Pressure Wax"=FALSE, "Spot Free Rinse"=FALSE, "Tire Shine Foam"=TRUE, "Air Dry"=FALSE, "Vehicle Out of Position"=FALSE} ("Car Wash Indicators")] -> w344
              tunnel: [w351 w355] -> w343
              tunnel: [TRUE w354] -> w342
              frame False {
                w351 = Controls."Tire Shine Foam"  # Next State
                # "Slider is out of position"
                n86 = call "Wash Timer.vi"("Operation"=enum16{"Init", "Read", "Pause"}."Pause") -> ("count"=w352:dbl)  [unwired: 10 in]
              }
              frame True {
                # "Slider in good position"
                n87 = call "Wash Timer.vi"("Operation"=enum16{"Init", "Read", "Pause"}."Read") -> ("count"=w358:dbl)  [unwired: 10 in]
                n88 = Greater Or Equal?(x=w358, y=5.0) -> (x >= y?=w356:bool)
                n89 = case shown="False" w356 {
                  tunnel: [w363 w365] -> w355
                  tunnel: [TRUE FALSE] -> w354
                  frame False {
                    w363 = Controls."Tire Shine Foam"  # Next State
                    # "5s not reached yet"
                  }
                  frame True {
                    # "5s is reached"
                    n90 = call "Steps Handler.vi"("Operation"=enum16{"Setup", "Next State"}."Next State") -> ("Next State"=w365:T3)  [unwired: 10 in]
                  }
                }
              }
            }
          }
        }
      }
      frame "Air Dry" {
        # "In good \nposition ?"
        # "In this state, we perform the \"Bug remover\" wash option. If it is in station 1, we read the timer.  Else, we pause the timer. \n\"Bug remover\" led is ON and \"Wash Entry\" is OFF. After 5s, we switch to next state."
        n91 = Equal?(x=w375, y=u8 3) -> (x = y?=w372:bool)
        n92 = case shown="True" w373 {
          tunnel: w372 -> [w381 w396]
          tunnel: [w380 w391] -> w371
          tunnel: [w379 w392] -> w370
          tunnel: [w378 w393] -> w369
          tunnel: [w377 w395] -> w368
          tunnel: [w376 w394] -> w367
          frame False {
            # "The wash option did not start yet because the slider is in the wrong position"
            n93 = case shown="True" w381 {
              tunnel: [_ TRUE] -> w380
              tunnel: [w384 w389] -> w379
              tunnel: [T2 {"Under Body Wash"=FALSE, "Bug Remover"=FALSE, "Pre-Soak"=FALSE, "High Pressure Wash"=FALSE, "Low Pressure Wax"=FALSE, "Spot Free Rinse"=FALSE, "Tire Shine Foam"=FALSE, "Air Dry"=FALSE, "Vehicle Out of Position"=TRUE} ("Car Wash Indicators") T2 {"Under Body Wash"=FALSE, "Bug Remover"=FALSE, "Pre-Soak"=FALSE, "High Pressure Wash"=FALSE, "Low Pressure Wax"=FALSE, "Spot Free Rinse"=FALSE, "Tire Shine Foam"=FALSE, "Air Dry"=TRUE, "Vehicle Out of Position"=FALSE} ("Car Wash Indicators")] -> w378
              tunnel: [_ w386] -> w377
              tunnel: [TRUE TRUE] -> w376
              frame False {
                w384 = Controls."Air Dry"  # Next State
                # "The slider is not in the good position!"
              }
              frame True {
                w389 = Controls."Air Dry"  # Next State
                # "In good position! We can initialize the timer."
                n94 = call "Wash Timer.vi"("Operation"=enum16{"Init", "Read", "Pause"}."Init") -> ("count"=w386:dbl)  [unwired: 10 in]
              }
            }
          }
          frame True {
            # "The wash option is ongoing"
            n95 = case shown="True" w396 {
              tunnel: [w401 w407] -> w395
              tunnel: [TRUE TRUE] -> w394
              tunnel: [T2 {"Under Body Wash"=FALSE, "Bug Remover"=FALSE, "Pre-Soak"=FALSE, "High Pressure Wash"=FALSE, "Low Pressure Wax"=FALSE, "Spot Free Rinse"=FALSE, "Tire Shine Foam"=FALSE, "Air Dry"=FALSE, "Vehicle Out of Position"=TRUE} ("Car Wash Indicators") T2 {"Under Body Wash"=FALSE, "Bug Remover"=FALSE, "Pre-Soak"=FALSE, "High Pressure Wash"=FALSE, "Low Pressure Wax"=FALSE, "Spot Free Rinse"=FALSE, "Tire Shine Foam"=FALSE, "Air Dry"=TRUE, "Vehicle Out of Position"=FALSE} ("Car Wash Indicators")] -> w393
              tunnel: [w400 w404] -> w392
              tunnel: [TRUE w403] -> w391
              frame False {
                w400 = Controls."Air Dry"  # Next State
                # "Slider is out of position"
                n96 = call "Wash Timer.vi"("Operation"=enum16{"Init", "Read", "Pause"}."Pause") -> ("count"=w401:dbl)  [unwired: 10 in]
              }
              frame True {
                # "Slider in good position"
                n97 = call "Wash Timer.vi"("Operation"=enum16{"Init", "Read", "Pause"}."Read") -> ("count"=w407:dbl)  [unwired: 10 in]
                n98 = Greater Or Equal?(x=w407, y=5.0) -> (x >= y?=w405:bool)
                n99 = case shown="False" w405 {
                  tunnel: [w412 w414] -> w404
                  tunnel: [TRUE FALSE] -> w403
                  frame False {
                    w412 = Controls."Air Dry"  # Next State
                    # "5s not reached yet"
                  }
                  frame True {
                    # "5s is reached"
                    n100 = call "Steps Handler.vi"("Operation"=enum16{"Setup", "Next State"}."Next State") -> ("Next State"=w414:T3)  [unwired: 10 in]
                  }
                }
              }
            }
          }
        }
      }
      frame "Exit" {
        # "In this state, we wait for the operator to place the Car Position Slider in the \"Exit\" position."
        # "In good \nposition ?"
        n101 = Equal?(x=w420, y=u8 4) -> (x = y?=w419:bool)
        n102 = case shown="False" w419 {
          tunnel: [w424 w425] -> w418
          tunnel: [T2 {"Under Body Wash"=FALSE, "Bug Remover"=FALSE, "Pre-Soak"=FALSE, "High Pressure Wash"=FALSE, "Low Pressure Wax"=FALSE, "Spot Free Rinse"=FALSE, "Tire Shine Foam"=FALSE, "Air Dry"=FALSE, "Vehicle Out of Position"=TRUE} ("Car Wash Indicators") _] -> w417
          tunnel: [TRUE _] -> w416
          frame False {
            w424 = Controls."Exit"  # Next State
            # "The Car Position Slider is not in the good position"
          }
          frame True {
            # "The Car Position Slider is in the good position"
            n103 = call "Steps Handler.vi"("Operation"=enum16{"Setup", "Next State"}."Next State") -> ("Next State"=w425:T3)  [unwired: 10 in]
          }
        }
      }
    }
    "Car Wash Indicators" <- w5
    "Wash Entry" <- w3
    "Elapsed Time" <- w4
    n104 = Wait (ms)(milliseconds to wait=u32 1) -> ()  [unwired: 1 out]
  }
